vi "Add Profile.vi"(8 "error in (no error)":errorcluster, 11 "Path":path) -> (0 "error out":errorcluster, 3 "Feedback":string)   [LabVIEW 2017]
doc: "Adds a WLAN profile to the specified interface on the computer."
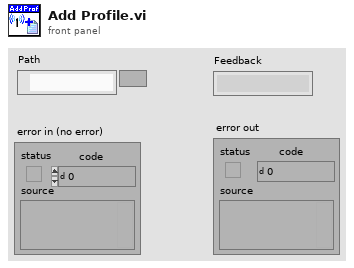
[diagram p1: front panel]
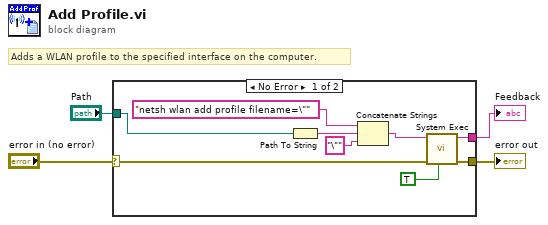
[diagram p0: block diagram]
diagram:
  # "Adds a WLAN profile to the specified interface on the computer."
  n1 = case shown="No Error" "error in (no error)" {
    selector: "error in (no error)" -> [w13 w14]
    tunnel: [w12 w14] -> w3
    tunnel: "Path" -> [w10 _]
    tunnel: [w6 _] -> w1
    frame No Error {
      n2 = Path To String(path=w10) -> (string=w9:string)
      n3 = Concatenate Strings("netsh wlan add profile filename=\"" ("string"), w9, "\"" ("string")) -> (w7:string)
      n4 = call <vilib>:"System Exec.vi"("run minimized? (F)"=TRUE, "error in (no error)"=w13, "command line"=w7) -> ("error out"=w12:errorcluster, "standard output"=w6:string)  [unwired: 5 in, 2 out]
    }
    frame Error {
    }
  }
  "error out" <- w3
  "Feedback" <- w1
